vi "Init SW Ring.vi"(8 "error in (no error)":errorcluster, 11 "[MV] Key Generator in":refnum<class "[MV] Key Generator.lvclass">) -> (0 "error out":errorcluster, 3 "[MV] Key Generator out":refnum<class "[MV] Key Generator.lvclass">)   [LabVIEW 2020, in "[MV] Key Generator.lvlib" / "[MV] Key Generator.lvclass"]
uses:
  [MV] Key Generator.lvclass
  [MV] Key Generator.lvclass/[MV] Key Generator.ctl
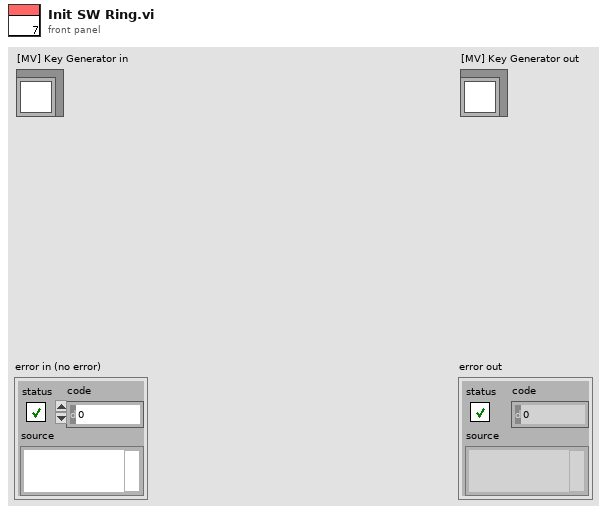
[diagram p1: front panel]
types:
  T1 = map{string, cluster{"private":string, "public":string}}
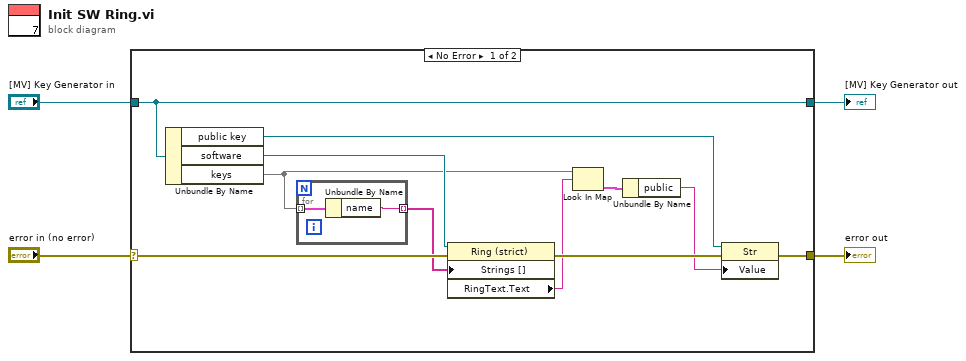
[diagram p0: block diagram]
diagram:
  n1 = case shown="No Error" "error in (no error)" {
    selector: "error in (no error)" -> [w15 w19]
    tunnel: [w6 w19] -> w3
    tunnel: [w13 w18] -> w1
    tunnel: "[MV] Key Generator in" -> [w13 w18]
    frame No Error {
      n2 = Unbundle By Name(w13) -> ("public key"=w10:refnum<vi>, "software"=w12:refnum<vi>, "keys"=w5:T1)
      n3 = for {
        tunnel: w5 -> [w17] mode=indexing
        tunnel: [w16] -> w14 mode=indexing
        n4 = Unbundle By Name(w17) -> ("name"=w16:string)
      }
      n5 = property class="Ring (strict)"(reference=w12, error in=w15, "Strings []"=w14) -> (error out=w11:errorcluster, "RingText.Text"=w9:string)  [unwired: 1 out]
      n6 = Look In Map(map=w5, key=w9) -> (value=w8:cluster{"private":string, "public":string})  [unwired: 1 in, 1 out]
      n7 = Unbundle By Name(w8) -> ("public"=w7:string)
      n8 = property class="Str"(reference=w10, error in=w11, "Value"=w7) -> (error out=w6:errorcluster)  [unwired: 1 out]
    }
    frame Error {
    }
  }
  "error out" <- w3
  "[MV] Key Generator out" <- w1
